vi "Read Stop Oven.vi"(8 "error in (no error)":errorcluster, 11 "Oven Actor in":refnum<class "Oven Actor.lvclass">) -> (0 "error out":errorcluster, 2 "Stop Oven":bool, 3 "Oven Actor out":refnum<class "Oven Actor.lvclass">)   [LabVIEW 2024, in "Oven Actor.lvlib" / "Oven Actor.lvclass"]
uses:
  Oven Actor.lvclass
  Oven Actor.lvclass/Oven Actor.ctl
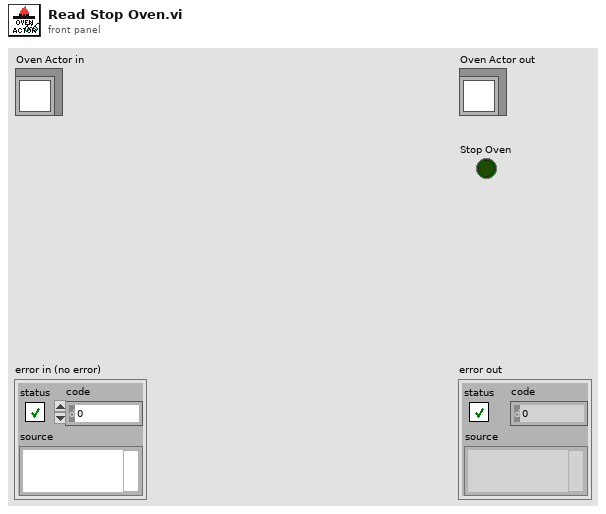
[diagram p1: front panel]
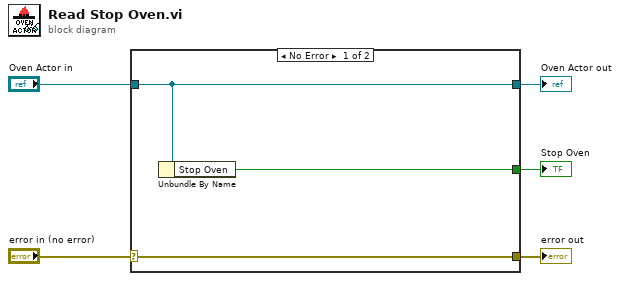
[diagram p0: block diagram]
diagram:
  n1 = case shown="No Error" "error in (no error)" {
    selector: "error in (no error)" -> [w8 w9]
    tunnel: [w8 w9] -> w4
    tunnel: [w7 w10] -> w2
    tunnel: "Oven Actor in" -> [w7 w10]
    tunnel: [w6 _] -> w1
    frame No Error {
      n2 = Unbundle By Name(w7) -> ("Stop Oven"=w6:bool)
    }
    frame Error {
    }
  }
  "error out" <- w4
  "Oven Actor out" <- w2
  "Stop Oven" <- w1
